vi "FTW-Event-Flatten.vi"(2 "UTC":bool, 7 "Event":T1 {"Timestamp" format="%<%Y-%m-%d %H:%M:%S%03u>T"; "Uptime" format="%.3ps"}) -> (8 "Flattened Event":string)   [LabVIEW 2015]
uses:
  FTW-Event.ctl
  Time/FTW-Time-DisplayFormat-Timestamp.ctl
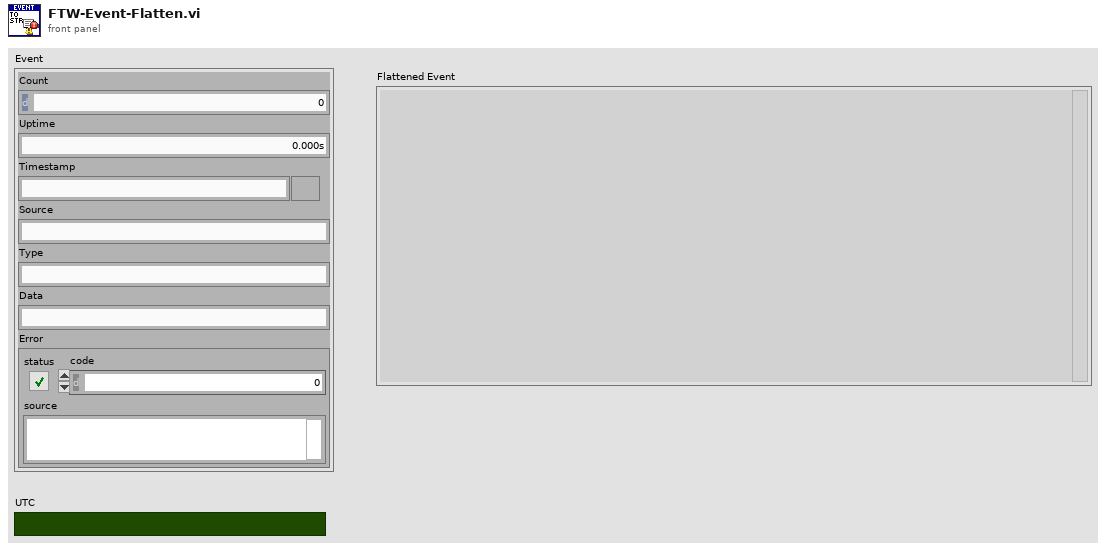
[diagram p1: front panel]
types:
  T1 = typedef "FTW-Event.ctl" = cluster{"Count":i32, "Uptime":dbl, "Timestamp":timestamp, "Source":string, "Type":string, "Data":string, "Error":errorcluster}
  T2 = typedef "FTW-Time-DisplayFormat-Timestamp.ctl" = enum16{"YYYY-MM-DDT00:00:00.000Z (UTC)", "YYYY-MM-DDT00:00:00.000 (locale)", "YYYY-MM-DDT00:00:00.000+hh:mm (time zone)", "YYYY-MM-DDT00-00-00Z (simple UTC)", "YYYY-MM-DDT00-00-00 (simple locale)", "YYYY-MM-DD"}
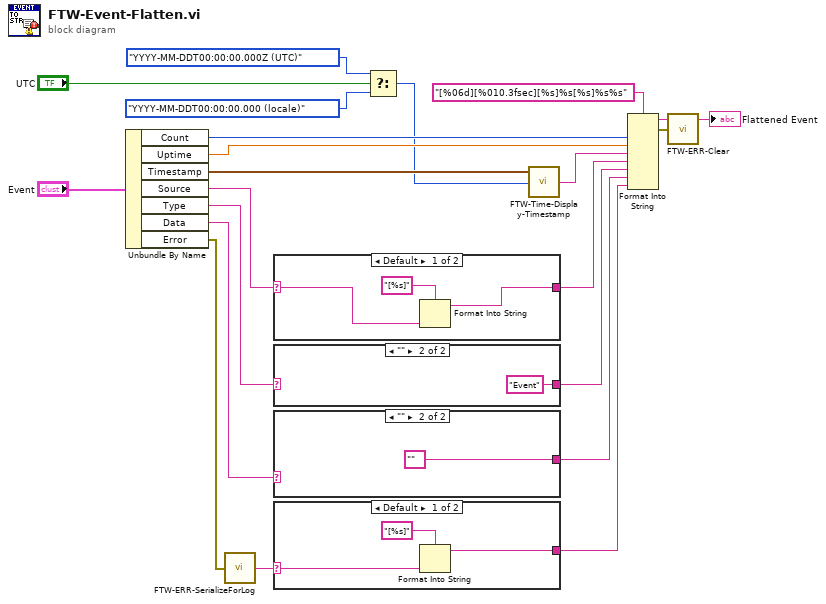
[diagram p0: block diagram]
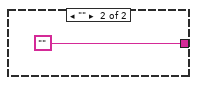
[diagram p2: hidden frame]
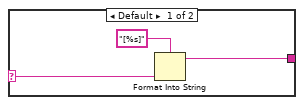
[diagram p4: hidden frame]
diagram:
  n1 = Unbundle By Name("Event") -> ("Count"=w13:i32, "Uptime"=w12:dbl, "Timestamp"=w6:timestamp, "Source"=w11:string, "Type"=w10:string, "Data"=w9:string, "Error"=w8:errorcluster)
  n2 = call "FTW-ERR-SerializeForLog.vi"("error in"=w8) -> ("Serialized Error"=w17:string)
  n3 = case shown="Default" w11 {
    selector: w11 -> [w23 w25]
    tunnel: [w22 w25] -> w14
    frame Default {
      n4 = Format Into String(format string="[%s]", w23) -> (resulting string=w22:string)  [unwired: 2 in, 1 out]
    }
    frame "" {
    }
  }
  n5 = case shown="\"\"" w10 {
    selector: w10 -> [w26 _]
    tunnel: [w26 "Event"] -> w15
    frame Default {
    }
    frame "" {
    }
  }
  n6 = case shown="\"\"" w9 {
    selector: w9 -> [w30 _]
    tunnel: [w29 ""] -> w19
    frame Default {
      n7 = Format Into String(format string="[%s]", w30) -> (resulting string=w29:string)  [unwired: 2 in, 1 out]
    }
    frame "" {
    }
  }
  n8 = case shown="Default" w17 {
    selector: w17 -> [w34 _]
    tunnel: [w33 ""] -> w16
    frame Default {
      n9 = Format Into String(format string="[%s]", w34) -> (resulting string=w33:string)  [unwired: 2 in, 1 out]
    }
    frame "" {
    }
  }
  n10 = Select(t=FTW-Time-DisplayFormat-Timestamp."YYYY-MM-DDT00:00:00.000Z (UTC)" ("Date Format"), s="UTC", f=FTW-Time-DisplayFormat-Timestamp."YYYY-MM-DDT00:00:00.000 (locale)" ("Date Format")) -> (s? t:f=w1:T2)
  n11 = call "FTW-Time-Display-Timestamp.vi"("Format"=w1, "Timestamp (unwired for current time)"=w6) -> ("Formatted Timestamp"=w5:string)  [unwired: 2 in]
  n12 = Format Into String(format string="[%06d][%010.3fsec][%s]%s[%s]%s%s", w13, w12, w5, w14, w15, w19, w16) -> (resulting string=→"Flattened Event":string, error out=w18:errorcluster)  [unwired: 2 in]
  n13 = call "FTW-ERR-Clear.vi"("error to snuff"=w18) -> ()  [unwired: 1 out]
